vi "listener.vi"() -> ()   [LabVIEW 2010]
doc: "OCW v3.0\n\nCopyright 2008 by Will Grover\n\nhttp://wgrover.com\n\nPermission is hereby granted, free of charge, to any person obtaining a copy of this software and associated documentation files (the \"Software\"), to deal in the Software without restriction, including without limitation the rights to use, copy, modify, merge, publish, distribute, sublicense, and/or sell copies of the Software, and to permit persons to whom the Software is furnished to do so, subject to the following conditions:\n\nThe above copyright notice and this permission notice shall be included in all copies or substantial portions of the Software.\n\nTHE SOFTWARE IS PROVIDED \"AS IS\", WITHOUT WARRANTY OF ANY KIND, EXPRESS OR IMPLIED, INCLUDING BUT NOT LIMITED TO THE WARRANTIES OF MERCHANTABILITY, FITNESS FOR A PARTICULAR PURPOSE AND NONINFRINGEMENT. IN NO EVENT SHALL THE AUTHORS OR COPYRIGHT HOLDERS BE LIABLE FOR ANY CLAIM, DAMAGES OR OTHER LIABILITY, WHETHER IN AN ACTION OF CONTRACT, TORT OR OTHERWISE, ARISING FROM, OUT OF OR IN CONNECTION WITH THE SOFTWARE OR THE USE OR OTHER DEALINGS IN THE SOFTWARE."
uses:
  <vilib>/DAQmx/write.llb/DAQmx Write (Digital Bool 1Line 1Point).vi
  <vilib>/Instr/_visa.llb/VISA Configure Serial Port (Instr).vi
  <vilib>/DAQmx/create/channels.llb/DAQmx Create Channel (DO-Digital Output).vi
  <vilib>/daqmx/miscellaneous.llb/DAQmx Fill In Error Info.vi
panel:
  in  "Lines":tag[](array[tag])=["Dev2/port0/line0", "Dev2/port0/line1", "Dev2/port0/line2", "Dev2/port0/line3", "Dev1/port0/line4", "Dev1/port0/line5", "Dev1/port0/line6", "Dev1/port0/line7", "Dev1/port0/line8", "Dev1/port0/line9", "Dev1/port0/line10", "Dev1/port0/line11", "Dev1/port0/line12", "Dev1/port0/line13", "Dev1/port0/line14", "Dev1/port0/line15"]
  # "Specify the digital lines you want to use.  The first line will be valve 0, the second line will be valve 1, and so on.  Drag the array to add or remove lines.\n\nWhen you are finished, remember to select\n\nEdit > Make Current Values Default \n\nfollowed by\n\nFile > Save\n\nso your selections will be remembered by the VI in the future.\n\nTo use this VI, simply run it and minimize the window.  This VI must be running to use manual.vi and ocw.vi."
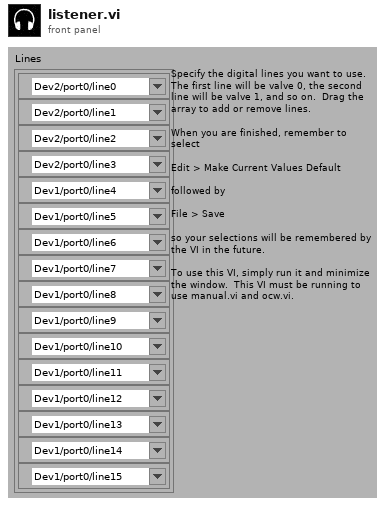
[diagram p1: front panel]
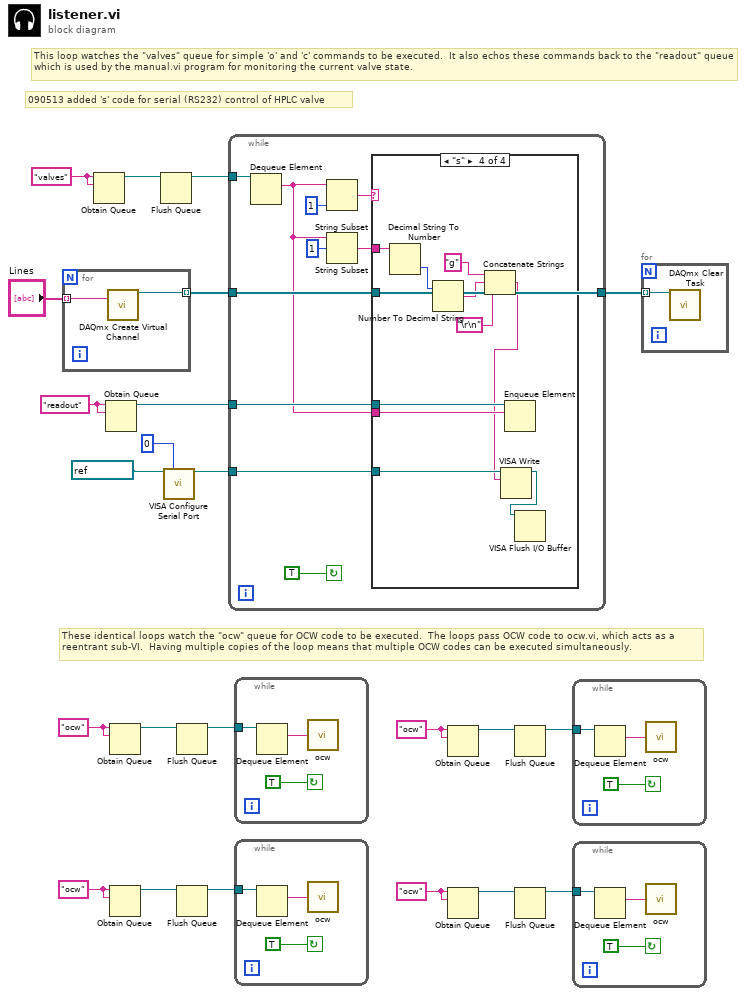
[diagram p0: block diagram]
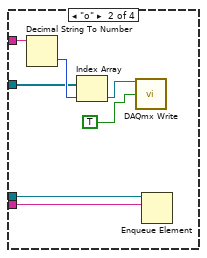
[diagram p3: hidden frame]
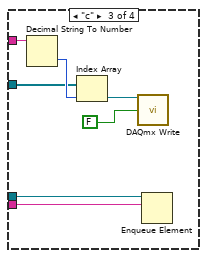
[diagram p4: hidden frame]
diagram:
  w6 = "ocw" ("name (unnamed)")
  w9 = "ocw" ("name (unnamed)")
  w12 = "ocw" ("name (unnamed)")
  w15 = "ocw" ("name (unnamed)")
  w16 = "readout" ("name (unnamed)")
  w20 = "valves" ("name (unnamed)")
  # "090513 added 's' code for serial (RS232) control of HPLC valve"
  # "This loop watches the \"valves\" queue for simple 'o' and 'c' commands to be executed.  It also echos these commands back to the \"readout\" queue which is used by the manual.vi program for monitoring the current valve state."
  # "These identical loops watch the \"ocw\" queue for OCW code to be executed.  The loops pass OCW code to ocw.vi, which acts as a reentrant sub-VI.  Having multiple copies of the loop means that multiple OCW codes can be executed simultaneously."
  n1 = for {
    tunnel: "Lines" -> [w25] mode=indexing
    tunnel: [w24] -> w21 mode=indexing
    n2 = call-poly <vilib>:"DAQmx Create Virtual Channel.vi"("lines"=w25) -> ("task out"=w24:refnum<k21>)  [unwired: 4 in, 10 out]
  }
  n3 = Obtain Queue(name (unnamed)=w20, element data type=w20) -> (queue out=w19:refnum<queue>)  [unwired: 3 in, 2 out]
  n4 = Obtain Queue(name (unnamed)=w16, element data type=w16) -> (queue out=w17:refnum<queue>)  [unwired: 3 in, 2 out]
  n5 = Obtain Queue(name (unnamed)=w15, element data type=w15) -> (queue out=w14:refnum<queue>)  [unwired: 3 in, 2 out]
  n6 = Obtain Queue(name (unnamed)=w12, element data type=w12) -> (queue out=w11:refnum<queue>)  [unwired: 3 in, 2 out]
  n7 = Flush Queue(queue=w19) -> (queue out=w18:refnum<queue>)  [unwired: 1 in, 2 out]
  n8 = call-poly "VISA Configure Serial Port"("VISA resource name"=refnum<visa-resource-name> "COM1", "timeout (10sec)"=u32 0) -> ("VISA resource name out"=w3:refnum<visa-resource-name>)  [unwired: 5 in, 8 out]
  n9 = Flush Queue(queue=w14) -> (queue out=w13:refnum<queue>)  [unwired: 1 in, 2 out]
  n10 = Flush Queue(queue=w11) -> (queue out=w10:refnum<queue>)  [unwired: 1 in, 2 out]
  n11 = while {
    tunnel: w18 -> [w30]
    tunnel: w21 -> [w31]
    tunnel: [w31] -> w22
    tunnel: w17 -> [w28]
    tunnel: w3 -> [w26]
    stop <- TRUE continue-if-true
    n12 = Dequeue Element(queue=w30) -> (element=w27:string)  [unwired: 1 in, 4 out]
    n13 = String Subset(string=w27, length (rest)=1 ("length (rest)")) -> (substring=w32:string)  [unwired: 1 out]
    n14 = String Subset(string=w27, offset (0)=1) -> (substring=w33:string)  [unwired: 1 out]
    n15 = case shown="\"s\"" w32 {
      tunnel: w33 -> [_ w41 w48 w59]
      tunnel: w31 -> [_ w40 w47 _]
      tunnel: w28 -> [_ w39 w44 w58]
      tunnel: w27 -> [_ w38 w43 w57]
      tunnel: w26 -> [_ _ _ w56]
      frame "", Default {
      }
      frame "o" {
        n16 = Decimal String To Number(string=w41) -> (number=w42:i32)  [unwired: 3 out]
        n17 = Index Array(array=w40, index=w42) -> (element=w37:refnum<k21>)
        n18 = call-poly <vilib>:"DAQmx Write.vi"("task/channels in"=w37, "data"=TRUE) -> ()  [unwired: 2 in, 12 out]
        n19 = Enqueue Element(queue=w39, element=w38) -> ()  [unwired: 1 in, 4 out]
      }
      frame "c" {
        n20 = Decimal String To Number(string=w48) -> (number=w49:i32)  [unwired: 3 out]
        n21 = Index Array(array=w47, index=w49) -> (element=w46:refnum<k21>)
        n22 = call-poly <vilib>:"DAQmx Write.vi"("task/channels in"=w46, "data"=FALSE) -> ()  [unwired: 2 in, 12 out]
        n23 = Enqueue Element(queue=w44, element=w43) -> ()  [unwired: 1 in, 4 out]
      }
      frame "s" {
        n24 = Decimal String To Number(string=w59) -> (number=w55:i32)  [unwired: 3 out]
        n25 = Number To Decimal String(number=w55) -> (decimal integer string=w53:string)  [unwired: 1 out]
        n26 = Concatenate Strings("g", w53, "\r\n") -> (w52:string)
        n27 = VISA Write(VISA resource name=w56, write buffer=w52) -> (VISA resource name out=w50:refnum<visa-resource-name>)  [unwired: 1 in, 2 out]
        n28 = Enqueue Element(queue=w58, element=w57) -> ()  [unwired: 1 in, 4 out]
        n29 = VISA Flush I/O Buffer(VISA resource name=w50) -> ()  [unwired: 1 in, 3 out]
      }
    }
  }
  n30 = while {
    tunnel: w13 -> [w61]
    stop <- TRUE continue-if-true
    n31 = Dequeue Element(queue=w61) -> (element=w60:string)  [unwired: 1 in, 4 out]
    n32 = call "ocw.vi"("in"=w60) -> ()  [unwired: 1 out]
  }
  n33 = while {
    tunnel: w10 -> [w64]
    stop <- TRUE continue-if-true
    n34 = Dequeue Element(queue=w64) -> (element=w63:string)  [unwired: 1 in, 4 out]
    n35 = call "ocw.vi"("in"=w63) -> ()  [unwired: 1 out]
  }
  n36 = Obtain Queue(name (unnamed)=w9, element data type=w9) -> (queue out=w8:refnum<queue>)  [unwired: 3 in, 2 out]
  n37 = Obtain Queue(name (unnamed)=w6, element data type=w6) -> (queue out=w5:refnum<queue>)  [unwired: 3 in, 2 out]
  n38 = Flush Queue(queue=w8) -> (queue out=w7:refnum<queue>)  [unwired: 1 in, 2 out]
  n39 = Flush Queue(queue=w5) -> (queue out=w4:refnum<queue>)  [unwired: 1 in, 2 out]
  n40 = while {
    tunnel: w7 -> [w67]
    stop <- TRUE continue-if-true
    n41 = Dequeue Element(queue=w67) -> (element=w66:string)  [unwired: 1 in, 4 out]
    n42 = call "ocw.vi"("in"=w66) -> ()  [unwired: 1 out]
  }
  n43 = while {
    tunnel: w4 -> [w70]
    stop <- TRUE continue-if-true
    n44 = Dequeue Element(queue=w70) -> (element=w69:string)  [unwired: 1 in, 4 out]
    n45 = call "ocw.vi"("in"=w69) -> ()  [unwired: 1 out]
  }
  n46 = for {
    tunnel: w22 -> [w72] mode=indexing
    n47 = call <vilib>:"DAQmx Clear Task.vi"("task in"=w72) -> ()  [unwired: 1 in, 14 out]
  }
